vi "Estructura_de_Casos.vi"() -> ()   [LabVIEW 2020]
panel:
  in  "Operaciones":enum16{"Suma", "Resta", "Mult", "Div"}(ring)
  out "Resultado":dbl
  in  "Num2":dbl
  in  "Num1":dbl
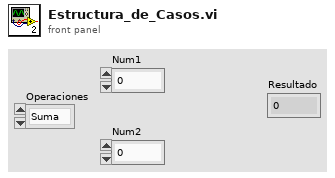
[diagram p1: front panel]
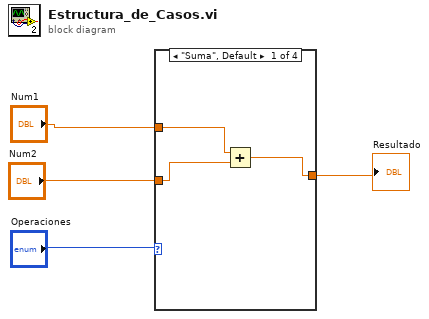
[diagram p0: block diagram]
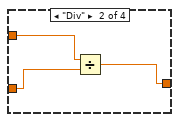
[diagram p2: hidden frame]
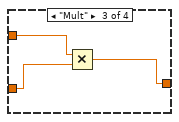
[diagram p3: hidden frame]
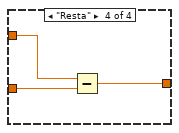
[diagram p4: hidden frame]
diagram:
  n1 = case shown="\"Suma\", Default" "Operaciones" {
    tunnel: "Num1" -> [w7 w10 w13 w16]
    tunnel: "Num2" -> [w6 w9 w12 w15]
    tunnel: [w5 w8 w11 w14] -> w1
    frame "Suma", Default {
      n2 = Add(x=w7, y=w6) -> (x+y=w5:dbl)
    }
    frame "Div" {
      n3 = Divide(x=w10, y=w9) -> (x/y=w8:dbl)
    }
    frame "Mult" {
      n4 = Multiply(x=w13, y=w12) -> (x*y=w11:dbl)
    }
    frame "Resta" {
      n5 = Subtract(x=w16, y=w15) -> (x-y=w14:dbl)
    }
  }
  "Resultado" <- w1
